vi "Inform.vi"(8 "error in (no error)":errorcluster, 10 "Message in":refnum<class "InformMessage.lvclass">, 11 "Waveform in":refnum<class "Waveform.lvclass">) -> (0 "error out":errorcluster, 3 "Waveform out":refnum<class "Waveform.lvclass">)   [LabVIEW 2012, in "Waveform.lvclass"]
doc: "The inform method processes the command inform'. \n\nThe command inform' is used for obtaining the latest instance data of the class. It also handles the current state of the observee and sets the 'ready' flag for the observee."
uses:
  Waveform.lvclass
  <vilib>/Distrio/Murmex/Murmex/Murmex.lvclass
  <vilib>/Distrio/Murmex/Message/Message.lvclass
  <vilib>/Distrio/Murmex/GenericMessage/GenericMessage.lvclass
  <vilib>/Distrio/Murmex/InformMessage/InformMessage.lvclass
panel:
  # "This method is called when the INFORM\ntrigger is sent. \n\nOverride this method when your component needs to\nrespond to this trigger. \n\nCall parent for proper implementation"
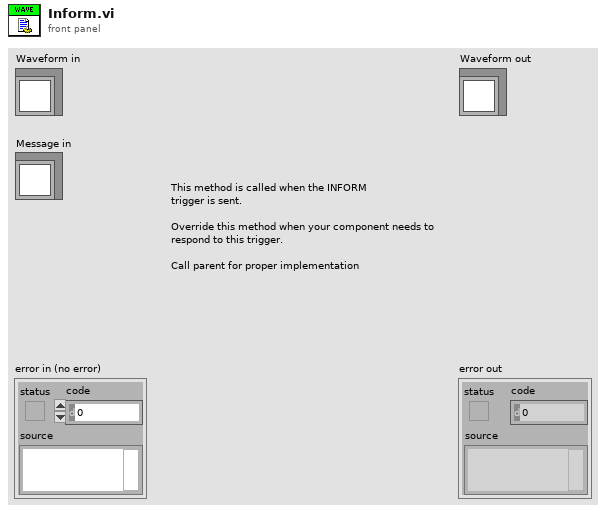
[diagram p1: front panel]
types:
  T1 = typedef "Murmex.lvlib/Murmex.lvclass/command_enum.ctl" = enum16{"null", "initialise", "reset", "terminate", "acknowledge", "update", "inspect", "inform", "proceed", "start", "stop", "fetch", "configure", "generic"}
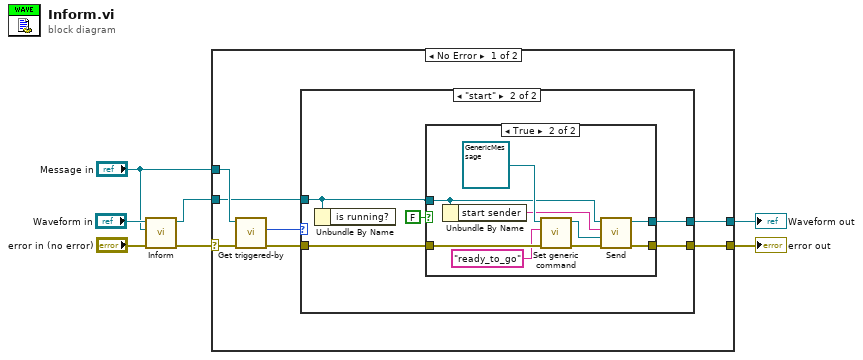
[diagram p0: block diagram]
diagram:
  n1 = call-parent "Inform.vi"("error in (no error)"="error in (no error)", "Message in"="Message in", "Murmex in"="Waveform in") -> ("error out"=w5:errorcluster, "Murmex out"=w4:refnum<class "Waveform.lvclass">)  [unwired: 7 in]
  n2 = case shown="No Error" w5 {
    selector: w5 -> [w14 w33]
    tunnel: w4 -> [w10 w34]
    tunnel: "Message in" -> [w13 _]
    tunnel: [w9 w33] -> w2
    tunnel: [w8 w34] -> w1
    frame No Error {
      n3 = call <vilib>:"Get triggered-by.vi"("error in (no error)"=w14, "Message in"=w13) -> ("error out"=w12:errorcluster, "triggered-by"=w11:T1)  [unwired: 7 in, 1 out]
      n4 = case shown="\"start\"" w11 {
        tunnel: w12 -> [w15 w21]
        tunnel: w10 -> [w16 w19]
        tunnel: [w15 w18] -> w9
        tunnel: [w16 w17] -> w8
        frame "null", Default {
        }
        frame "start" {
          n5 = Unbundle By Name(w19) -> ()  [unwired: 1 out]
          n6 = case shown="True" FALSE {
            tunnel: w21 -> [w22 w32]
            tunnel: w19 -> [w23 w27]
            tunnel: [w22 w25] -> w18
            tunnel: [w23 w24] -> w17
            frame False {
            }
            frame True {
              n7 = Unbundle By Name(w27) -> ("start sender"=w26:string)
              n8 = call <vilib>:"Set generic command.vi"("error in (no error)"=w32, "generic command"="ready_to_go", "GenericMessage in"=refnum<class "GenericMessage.lvclass"> refnum ("Message in")) -> ("error out"=w29:errorcluster, "GenericMessage out"=w28:refnum<class "GenericMessage.lvclass">)  [unwired: 7 in]
              n9 = call <vilib>:"Send.vi"("error in (no error)"=w29, "Message"=w28, "recipient"=w26, "Murmex in"=w27) -> ("error out"=w25:errorcluster, "Murmex out"=w24:refnum<class "Waveform.lvclass">)  [unwired: 6 in]
            }
          }
        }
      }
    }
    frame Error {
    }
  }
  "error out" <- w2
  "Waveform out" <- w1
